vi "Preprocess DataSockets.vi"(8 "error in (no error)":errorcluster, 11 "Response Synchronizer in":refnum<class "Response Synchronizer.lvclass">) -> (0 "error out":errorcluster, 3 "Response Synchronizer out":refnum<class "Response Synchronizer.lvclass">)   [LabVIEW 2021, in "Response Synchronizer.lvclass"]
uses:
  Response Synchronizer.lvclass
  Response Synchronizer.lvclass/Response Synchronizer.ctl
  NHMFL_Core/Libraries/Instruments/Results/Acquired Result/Acquired Result.lvclass
  <vilib>/express/express signal manip/GetorSetDDTAttributes/Set DDT Attributes/Set DDT Properties.xnode
  <vilib>/express/express shared/transition.llb/Dynamic To Waveform Array.vi
  <vilib>/express/express signal manip/GetorSetDDTAttributes/Set DDT Attributes/SetT0.vi
  <vilib>/express/express shared/transition.llb/Waveform Array To Dynamic.vi
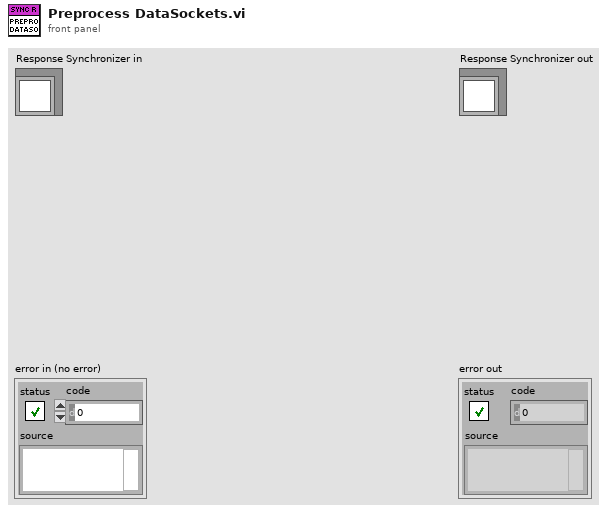
[diagram p1: front panel]
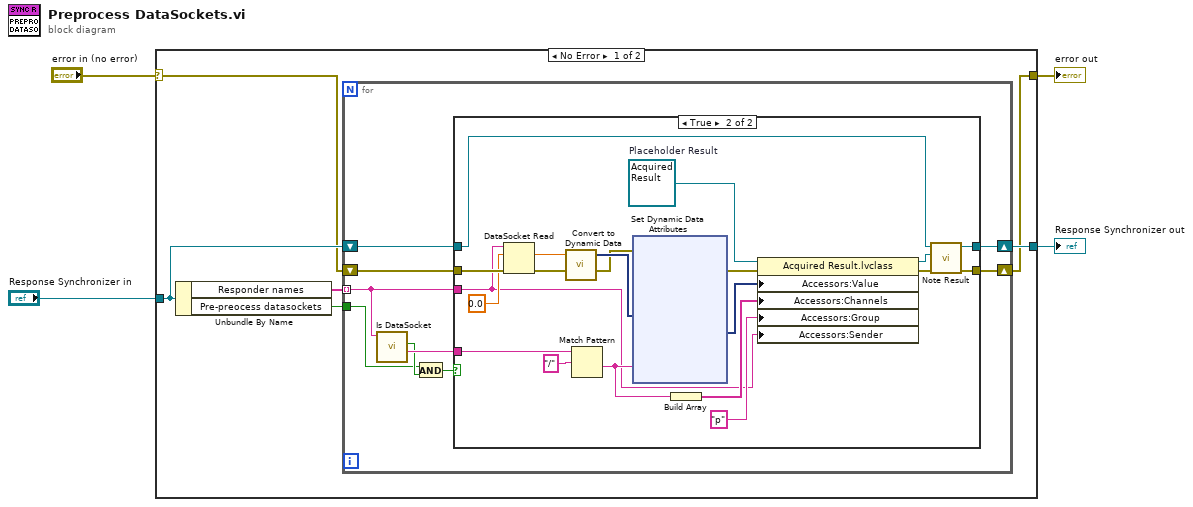
[diagram p0: block diagram]
diagram:
  n1 = case shown="No Error" "error in (no error)" {
    selector: "error in (no error)" -> [w6 w56]
    tunnel: [w5 w56] -> w3
    tunnel: [w10 w55] -> w1
    tunnel: "Response Synchronizer in" -> [w9 w55]
    frame No Error {
      n2 = Unbundle By Name(w9) -> ("Responder names"=w8:string[], "Pre-preocess datasockets"=w7:bool)
      n3 = for {
        tunnel: w7 -> [w13]
        tunnel: w8 -> [w16] mode=indexing
        shift-right: [w17] -> w5
        shift-left: w6 -> [w18]
        shift-right: [w11] -> w10
        shift-left: w9 -> [w12]
        n4 = call "Is DataSocket.vi"("String"=w16) -> ("After header"=w15:string, "DataSocket"=w14:bool)  [unwired: 9 in]
        n5 = And(x=w13, y=w14) -> (x .and. y?=w19:bool)
        n6 = case shown="True" w19 {
          tunnel: w16 -> [_ w22]
          tunnel: w18 -> [w21 w40]
          tunnel: [w21 w27] -> w17
          tunnel: [w20 w25] -> w11
          tunnel: w15 -> [_ w32]
          tunnel: w12 -> [w20 w24]
          frame False {
          }
          frame True {
            w23 = refnum<class "Acquired Result.lvclass"> refnum  # Placeholder Result
            n7 = DataSocket Read(8:w40, 10:0.0 ("DBL Value"), 11:w22) -> (0:w35:errorcluster, 2:w36:dbl)  [unwired: 2 in, 5 out]
            n8 = call "Convert to Dynamic Data"("Double"=w36) -> ("Dynamic Data Type"=w37:dynamicdata)  [unwired: 3 in]
            n9 = Match Pattern(string=w32, regular expression="/") -> (after substring=w30:string)  [unwired: 1 in, 3 out]
            n10 = xnode "Set Dynamic Data Attributes"("Signals In"=w37, "Signal Name"=w30, "error in"=w35) -> ("Signals Out"=w33:dynamicdata, "error out"=w34:errorcluster)  [unwired: 1 in]
            n11 = Build Array(w30) -> (w29:string[])
            n12 = property class="Acquired Result.lvclass"(reference=w23, error in=w34, "Accessors:Value"=w33, "Accessors:Channels"=w29, "Accessors:Group"="p" ("Group"), "Accessors:Sender"=w22) -> (reference out=w26:refnum<class "Acquired Result.lvclass">, error out=w39:errorcluster)
            n13 = call-dynamic "Note Result.vi"("error in (no error)"=w39, "Acquired Result.lvclass"=w26, "Response Synchronizer in"=w24) -> ("error out"=w27:errorcluster, "Response Synchronizer out"=w25:refnum<class "Response Synchronizer.lvclass">)  [unwired: 7 in]
          }
        }
      }
    }
    frame Error {
    }
  }
  "error out" <- w3
  "Response Synchronizer out" <- w1
